vi "ZC_gouru.vi"(0 "action":string, 1 "LabVIEW Web Service Request":refnum<class "Web Request.lvclass"> caption="LabVIEW Web服务请求", 3 "hetong":string, 4 "beizhu":string, 5 "id":string, 6 "didian":string, 7 "number_base":string, 11 "number":string, 14 "status":string, 15 "key":string) -> (10 "error":errorcluster)   [LabVIEW 2017]
uses:
  <vilib>/wsapi/Web Request.lvclass
panel:
  out "postdata":string caption="post数据"
  out "error out":errorcluster caption="错误输出"
  # "Web服务请求输入接线端用于调用“Web服务”选板的VI。除非不需要访问该选板，否则不要在连线板上删除这个输入接线端。"
  # "添加至连线板的每一个其他输入控件，在URL中对应于一个输入。如需在接线端模式输出（默认设置）下包含显示控件，则该显示控件必须与连线板相连。"
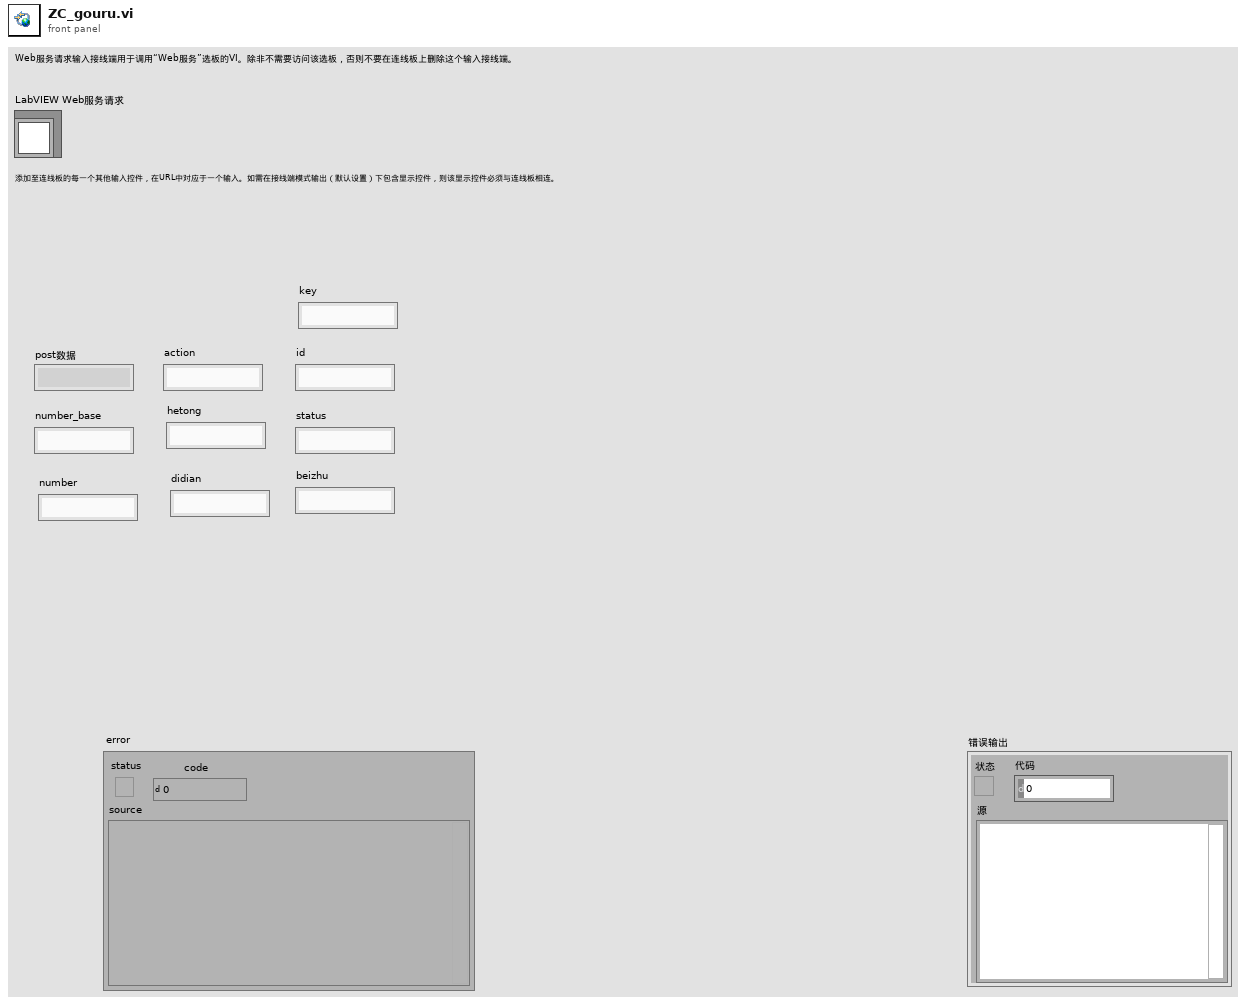
[diagram p1: front panel]
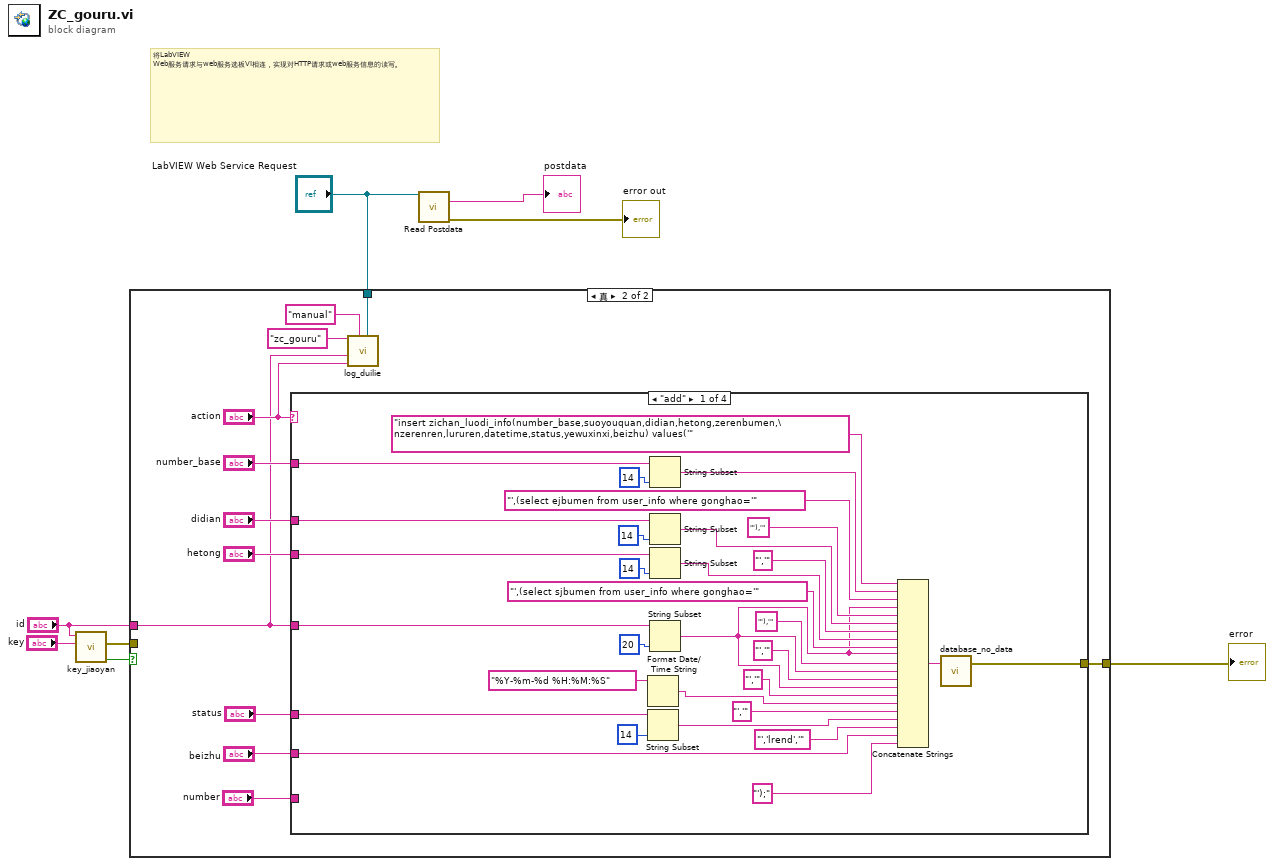
[diagram p0: block diagram]
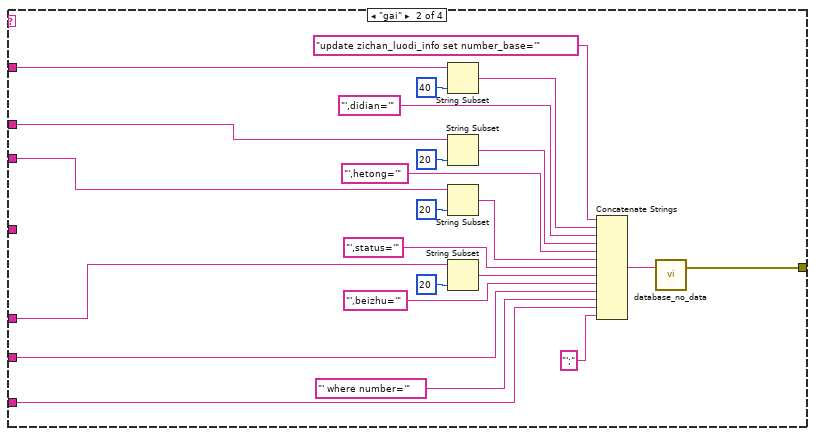
[diagram p3: hidden frame]
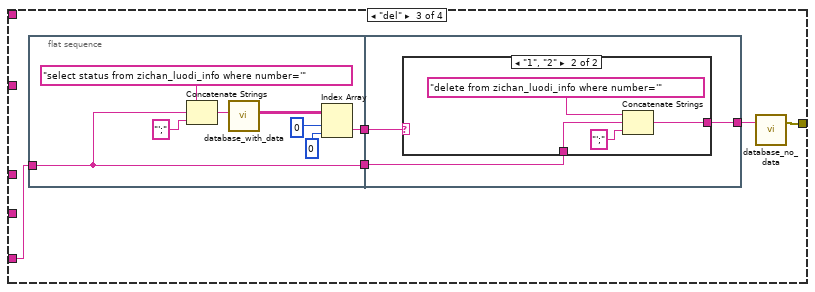
[diagram p4: hidden frame]
diagram:
  # "将LabVIEW Web服务请求与web服务选板VI相连，实现对HTTP请求或web服务信息的读写。"
  n1 = call "key_jiaoyan.vi"("key_client"="key", "gonghao"="id") -> ("jy"=w2:bool, "error"=w1:errorcluster)  [unwired: 8 in]
  n2 = case shown="真" w2 {
    tunnel: [w9 w21] -> w7
    tunnel: "LabVIEW Web Service Request" -> [_ w12]
    tunnel: "id" -> [_ w10]
    tunnel: w1 -> [w9 _]
    frame False {
    }
    frame True {
      n3 = case shown="\"add\"" "action" {
        tunnel: [w33 w53 w76 _] -> w21
        tunnel: "didian" -> [w32 w59 _ _]
        tunnel: w10 -> [w31 _ _ _]
        tunnel: "hetong" -> [w30 w58 _ _]
        tunnel: "number_base" -> [w29 w60 _ _]
        tunnel: "status" -> [w28 w57 _ _]
        tunnel: "beizhu" -> [w27 w56 _ _]
        tunnel: "number" -> [_ w55 w78 _]
        frame "add" {
          n4 = Format Date/Time String(time format string (%c)="%Y-%m-%d %H:%M:%S" ("时间格式字符串(%c)")) -> (date/time string=w22:string)  [unwired: 2 in]
          n5 = String Subset(string=w28, length (rest)=14 ("长度（剩余）")) -> (substring=w41:string)  [unwired: 1 in]
          n6 = String Subset(string=w29, length (rest)=14 ("长度（剩余）")) -> (substring=w50:string)  [unwired: 1 in]
          n7 = String Subset(string=w32, length (rest)=14 ("长度（剩余）")) -> (substring=w38:string)  [unwired: 1 in]
          n8 = String Subset(string=w30, length (rest)=14 ("长度（剩余）")) -> (substring=w48:string)  [unwired: 1 in]
          n9 = String Subset(string=w31, length (rest)=20 ("长度（剩余）")) -> (substring=w23:string)  [unwired: 1 in]
          n10 = Concatenate Strings("insert zichan_luodi_info(number_base,suoyouquan,didian,hetong,zerenbumen,\nzerenren,lururen,datetime,status,yewuxinxi,beizhu) values('" ("格式字符串"), w50, "',(select ejbumen from user_info where gonghao='" ("字符串"), w23, "'),'" ("字符串"), w38, "','" ("字符串"), w48, "',(select sjbumen from user_info where gonghao='" ("字符串"), w23, "'),'" ("字符串"), w23, "','" ("字符串"), w23, "','" ("字符串"), w22, "','" ("字符串"), w41, "','lrend','" ("字符串"), w27, "');" ("字符串")) -> (w34:string)
          n11 = call "database_no_data.vi"("input"=w34) -> ("error"=w33:errorcluster)  [unwired: 2 in]
        }
        frame "gai" {
          n12 = String Subset(string=w60, length (rest)=40 ("长度（剩余）")) -> (substring=w71:string)  [unwired: 1 in]
          n13 = String Subset(string=w59, length (rest)=20 ("长度（剩余）")) -> (substring=w69:string)  [unwired: 1 in]
          n14 = String Subset(string=w58, length (rest)=20 ("长度（剩余）")) -> (substring=w67:string)  [unwired: 1 in]
          n15 = String Subset(string=w57, length (rest)=20 ("长度（剩余）")) -> (substring=w65:string)  [unwired: 1 in]
          n16 = Concatenate Strings("update zichan_luodi_info set number_base='" ("格式字符串"), w71, "',didian='" ("字符串"), w69, "',hetong='" ("字符串"), w67, "',status='" ("字符串"), w65, "',beizhu='" ("字符串"), w56, "' where number='" ("字符串"), w55, "';" ("字符串")) -> (w54:string)
          n17 = call "database_no_data.vi"("input"=w54) -> ("error"=w53:errorcluster)  [unwired: 2 in]
        }
        frame "del" {
          n18 = flat-sequence {
            tunnel: w78 -> [w86]
            tunnel: [w86] -> w80
            tunnel: [w81] -> w79
            tunnel: [w91] -> w77
            tunnel: w80 -> [w90]
            tunnel: w79 -> [w89]
            frame #0 {
              n19 = Concatenate Strings("select status from zichan_luodi_info where number='" ("格式字符串"), w86, "';" ("字符串")) -> (w85:string)
              n20 = call "database_with_data.vi"("input"=w85) -> ("Data"=w82:string[][])  [unwired: 9 in, 1 out]
              n21 = Index Array(array=w82, index (row)=0 ("索引 (行)"), index (col)=0 ("禁用的索引 (列)")) -> (element=w81:string)
            }
            frame #1 {
              n22 = case shown="\"1\", \"2\"" w89 {
                tunnel: [_ w93] -> w91
                tunnel: w90 -> [_ w92]
                frame "假", Default {
                }
                frame "1", "2" {
                  n23 = Concatenate Strings("delete from zichan_luodi_info where number='" ("格式字符串"), w92, "';" ("字符串")) -> (w93:string)
                }
              }
            }
          }
          n24 = call "database_no_data.vi"("input"=w77) -> ("error"=w76:errorcluster)  [unwired: 2 in]
        }
        frame Default {
        }
      }
      n25 = call "log_duilie.vi"("LabVIEW Web Service Request"=w12, "type"="manual", "action"="action", "user"=w10, "yw"="zc_gouru") -> ()  [unwired: 7 in]
    }
  }
  "error" <- w7
  n26 = call <vilib>:"Read Postdata.vi"("LabVIEW Web Service Request"="LabVIEW Web Service Request") -> ("postdata"=→"postdata":string, "error out"=→"error out":errorcluster)  [unwired: 12 in, 1 out]
